vi "ApplyColorGain.vi"(10 "Gain":dbl, 11 "Color In":u32) -> (3 "Color Out":u32)   [LabVIEW 2020, in "ArduinoSerialBling.lvlib"]
uses:
  ArduinoSerialBling.lvlib
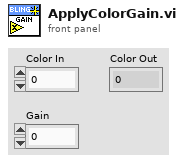
[diagram p1: front panel]
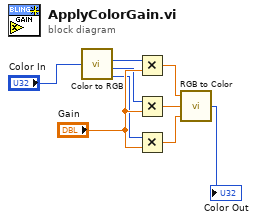
[diagram p0: block diagram]
diagram:
  n1 = call <vilib>:"Color to RGB.vi"("Color"="Color In") -> ("R"=w3:u8, "G"=w2:u8, "B"=w1:u8)  [unwired: 1 out]
  n2 = Multiply(x=w3, y="Gain") -> (x*y=w6:dbl)
  n3 = Multiply(x=w2, y="Gain") -> (x*y=w7:dbl)
  n4 = Multiply(x=w1, y="Gain") -> (x*y=w8:dbl)
  n5 = call <vilib>:"RGB to Color.vi"("B"=w8, "G"=w7, "R"=w6) -> ("Color"=→"Color Out":u32)
